vi "Tracking Test Teleop.vi"(10 "Match Info":T1={"Autonomous Elapsed Seconds"=0.0, "TeleOp Elapsed Seconds"=0.0, "Disabled Elapsed Seconds"=0.0, "Visited Autonomous"=FALSE, "Visited TeleOp"=FALSE, "Visited Disabled"=FALSE, "Autonomous Settings"={"Autonomous Style"=enum."Independent", "VI Refnum"=refnum}}, 11 "Call Context":T2) -> ()   [LabVIEW 2020]
doc: "This VI is called for each TeleOp packet received from the DS where the robot is not disabled. It is often used to read from the joysticks and update I/O or to update setpoints for timed control loops. It should complete and return within 20 milliseconds or it may miss DS packets."
uses:
  <vilib>/Rock Robotics/Network Tables/NT Write Boolean.vi
  Systems/Game Controller/Global_SEN_Data Out.vi
  Systems/Game Controller/GameController_SEN.lvlib
  Systems/SwerveDrive/Global_CMD_ACT_Data In.vi
  Systems/SwerveDrive/SwerveDrive_ACT.lvlib
  Shared Code/TypeDefs/ENUM_Swerve_CMD_Mode Select.ctl
  Shared Code/TypeDefs/Cluster_CMD_Direction Data.ctl
  Systems/SwerveDrive/Cluster_CMD_ACT_Data.ctl
  Shared Code/TypeDefs/Dial_Compase heading unit circle CCW positive.ctl
  Shared Code/TypeDefs/Level_Velocity plus-minus 1.ctl
  Shared Code/TypeDefs/Cluster_Module Velocity-Direction-Rotations.ctl
  Shared Code/TypeDefs/Cluster_X-Y.ctl
  <vilib>/Rock Robotics/WPI/ThirdParty/PhotonVisionLib/PhotonVisionLib.lvlib
  Type Defs/NUM_Rotate Input.ctl
  <vilib>/Rock Robotics/WPI/DriverStation/WPI_DriverStationMatch Info.ctl
  <vilib>/Rock Robotics/WPI/DriverStation/WPI_DriverStationDerivedRobotMode.ctl
panel:
  out "Rotation":dbl
  in  "Camera Pitch(deg)":dbl
  in  "TargetHeight_Meters":dbl=1.5
  in  "CameraHeight_Meters":dbl
  in  "CameraName":string="main"
  in  "Enabled":bool
  in  "Translation Speed (ft/s)":dbl=10.0 format="%#_13g"
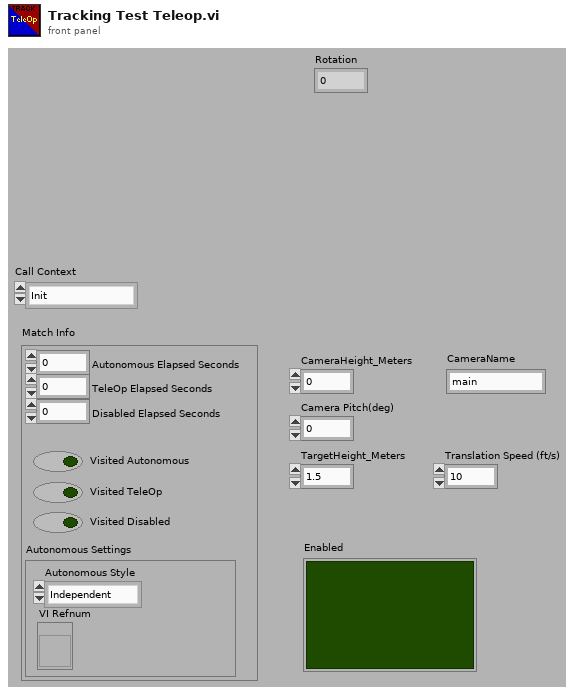
[diagram p1: front panel]
types:
  T1 = typedef "WPI_DriverStationMatch Info.ctl" = cluster{"Autonomous Elapsed Seconds":dbl, "TeleOp Elapsed Seconds":dbl, "Disabled Elapsed Seconds":dbl, "Visited Autonomous":bool, "Visited TeleOp":bool, "Visited Disabled":bool, "Autonomous Settings":cluster{"Autonomous Style":enum16{"Iterative", "Independent"}, "VI Refnum":refnum<vi>}}
  T2 = typedef "WPI_DriverStationDerivedRobotMode.ctl" = enum16{"Init", "Execute", "Stop"}
  T3 = typedef "Cluster_X-Y.ctl" = cluster{"X":dbl, "Y":dbl}
  T4 = typedef "ENUM_Swerve_CMD_Mode Select.ctl" = enum16{"Stop", "Move", "Turret Manual"}
  T5 = typedef "Cluster_Module Velocity-Direction-Rotations.ctl" = cluster{"Velocity":T6, "Angle":T7, "Rotations Count":dbl}
  T6 = typedef "Level_Velocity plus-minus 1.ctl" = dbl
  T7 = typedef "Dial_Compase heading unit circle CCW positive.ctl" = dbl
  T8 = typedef "SwerveDrive_ACT.lvlib/Cluster_CMD_ACT_Data.ctl" = cluster{"Mode":T4, "Direction":T9, "Orientation Robot(t) Field(f)":bool, "Max Translation Speed (ft/sec)":dbl, "Rotation Reduction 1-0":dbl, "Rotation Center From Robot Center":T3}
  T9 = typedef "Cluster_CMD_Direction Data.ctl" = cluster{"Traverse":T5, "Rotate(Yaw) CCW 1 CW -1":T10}
  T10 = typedef "NUM_Rotate Input.ctl" = dbl
  T11 = typedef "PhotonVisionLib.lvlib/PhotonPipelineResultType.ctl" = cluster{"TargetCount":i32, "Latency_MilliSec":dbl, "Targets":T12[]}
  T12 = typedef "PhotonVisionLib.lvlib/PhotonTrackedTargetType.ctl" = cluster{"Yaw":dbl, "Pitch":dbl, "Area":dbl, "Skew":dbl, "TargetCorners":T13[], "CameraToTarget":T14}
  T13 = typedef "PhotonVisionLib.lvlib/TargetCornerType.ctl" = cluster{"X":dbl, "Y":dbl}
  T14 = typedef "Trajectory_Library.lvlib/TRANSFORM2D.ctl" = cluster{"TRANSLATION":T15, "ROTATION":T16}
  T15 = typedef "Trajectory_Library.lvlib/TRANSLATION2D.ctl" = cluster{"X":dbl, "Y":dbl}
  T16 = typedef "Trajectory_Library.lvlib/ROTATION2D.ctl" = cluster{"VALUE":dbl, "COS":dbl, "SIN":dbl}
  T17 = typedef "Trajectory_Library.lvlib/ROTATION3D.ctl" = cluster{"Q_quaternion":T18}
  T18 = typedef "Trajectory_Library.lvlib/QUATERNION.ctl" = cluster{"R":dbl, "V":dbl[]}
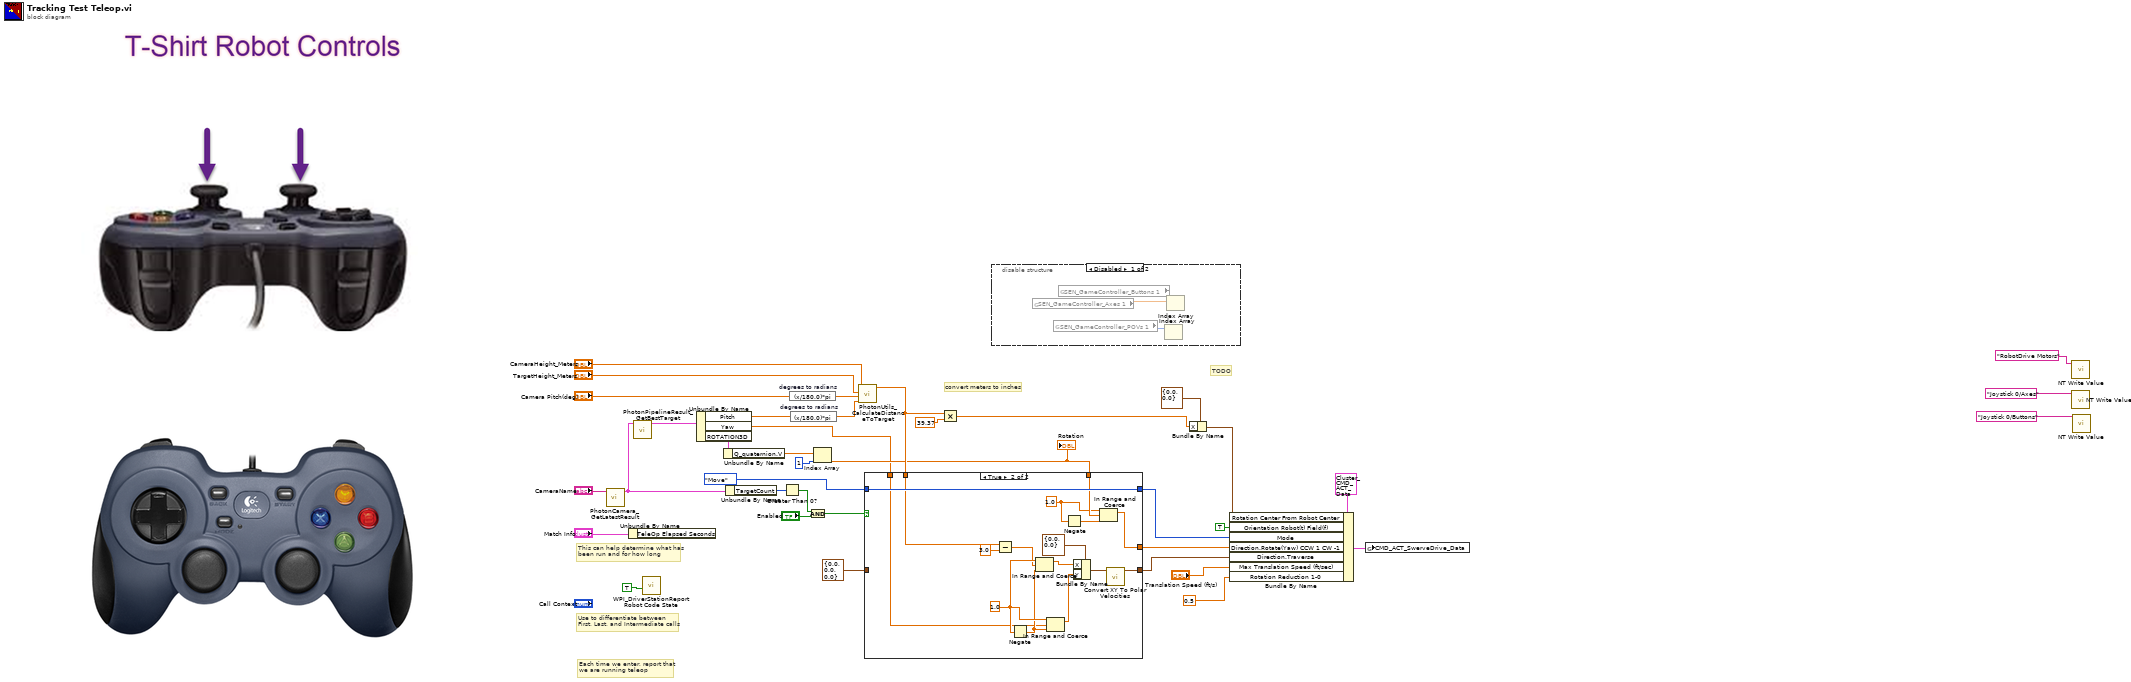
[diagram p0: block diagram]
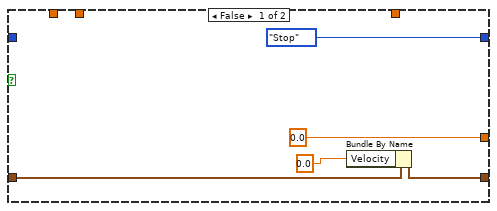
[diagram p2: hidden frame]
diagram:
  # "convert meters to inches"
  # "TODO"
  # "Each time we enter, report that\nwe are running teleop"
  # "Use to differentiate between\nFirst, Last, and Intermediate calls"
  # "This can help determine what has\nbeen run and for how long"
  n1 = call <vilib>:"PhotonCamera_GetLatestResult.vi"("CameraName"="CameraName") -> ("PipelineResult"=w19:T11)  [unwired: 9 in, 1 out]
  n2 = Unbundle By Name("Match Info") -> ()  [unwired: 1 out]
  n3 = call <vilib>:"PhotonPipelineResult_GetBestTarget.vi"("PhotonPipelineResult"=w19) -> ("PhotonTrackedTarget"=w6:T12)  [unwired: 10 in]
  n4 = call <vilib>:"WPI_DriverStationReport Robot Code State.vi"("TeleOp"=TRUE ("Autonomous")) -> ()  [unwired: 10 in, 1 out]
  n5 = Unbundle By Name(w6) -> ("Pitch"=w11:dbl, "Yaw"=w1:dbl, "ROTATION3D"=w4:T17)
  n6 = Unbundle By Name(w4) -> ("Q_quaternion.V"=w3:dbl[])
  n7 = Unbundle By Name(w19) -> ("TargetCount"=w23:i32)
  n8 = Greater Than 0?(x=w23) -> (x > 0?=w22:bool)
  n9 = expression code="(x/180.0)*pi" "degrees to radians"("Camera Pitch(deg)") -> (w15:dbl)
  n10 = expression code="(x/180.0)*pi" "degrees to radians"(w11) -> (w14:dbl)
  n11 = And(x=w22, y="Enabled") -> (x .and. y?=w20:bool)
  n12 = Index Array(array=w3, index=1) -> (element=w2:dbl)
  "Rotation" <- w2
  n13 = call <vilib>:"PhotonUtils_CalculateDistanceToTarget.vi"("TargetPitch_Radians"=w14, "CameraPitch_Radians"=w15, "TargetHeight_Meters"="TargetHeight_Meters", "CameraHeight_Meters"="CameraHeight_Meters") -> ("DistanceToTarget_Meters"=w9:dbl)  [unwired: 7 in]
  n14 = case shown="True" w20 {
    tunnel: ENUM_Swerve_CMD_Mode_Select."Move" ("Mode") -> [_ w59]
    tunnel: [ENUM_Swerve_CMD_Mode_Select."Stop" ("Mode") w59] -> w33
    tunnel: T5 {"Velocity"=0.0, "Angle"=0.0, "Rotations Count"=0.0} ("Polar Out") -> [w41 _]
    tunnel: [w42 w56] -> w29
    tunnel: w9 -> [_ w49]
    tunnel: w1 -> [_ w48]
    tunnel: [0.0 ("f") w44] -> w7
    tunnel: w2 -> [_ w47]
    frame False {
      n15 = Bundle By Name(cluster=w41, "Velocity"=T6 0.0) -> (w42:T5)
    }
    frame True {
      w45 = 1.0 ("upper limit")
      w54 = 1.0 ("upper limit")
      n16 = Subtract(x=w49, y=3.0) -> (x-y=w52:dbl)
      n17 = Negate(x=w54) -> (-x=w53:dbl)
      n18 = In Range and Coerce(upper limit=w54, x=w52, lower limit=w53) -> (coerced(x)=w51:dbl)  [unwired: 1 out]
      n19 = In Range and Coerce(upper limit=w54, x=w48, lower limit=w53) -> (coerced(x)=w50:dbl)  [unwired: 1 out]
      n20 = Negate(x=w45) -> (-x=w46:dbl)
      n21 = Bundle By Name(cluster=T3 {"X"=0.0, "Y"=0.0} ("XY Velocities"), "X"=w51, "Y"=w50) -> (w58:T3)
      n22 = In Range and Coerce(upper limit=w45, x=w47, lower limit=w46) -> (coerced(x)=w44:dbl)  [unwired: 1 out]
      n23 = call "Convert XY To Polar Velocities.vi"("XY Velocities"=w58) -> ("Polar Out"=w56:T5)  [unwired: 10 in]
    }
  }
  n24 = Multiply(x=w9, y=39.37) -> (x*y=w8:dbl)
  n25 = disable-structure shown="Disabled" {
    frame Disabled {
      n26 = global read "Global_SEN_Data Out.vi" "SEN_GameController_Axes 1"() -> (w61:dbl[])
      n27 = global read "Global_SEN_Data Out.vi" "SEN_GameController_POVs 1"() -> (w60:i16[])
      n28 = global read "Global_SEN_Data Out.vi" "SEN_GameController_Buttons 1"() -> ()  [unwired: 1 out]
      n29 = Index Array(array=w60) -> ()  [unwired: 1 in, 1 out]
      n30 = Index Array(array=w61) -> ()  [unwired: 1 in, 1 out]
    }
    frame Enabled {
    }
  }
  n31 = Bundle By Name(cluster=T3 {"X"=0.0, "Y"=0.0} ("Rotation Center From Robot Center"), "X"=w8) -> (w17:T3)
  n32 = Bundle By Name(cluster=T8 {"Mode"=enum."Stop", "Direction"={"Traverse"={"Velocity"=0.0, "Angle"=0.0, "Rotations Count"=0.0}, "Rotate(Yaw) CCW 1 CW -1"=0.0}, "Orientation Robot(t) Field(f)"=FALSE, "Max Translation Speed (ft/sec)"=0.0, "Rotation Reduction 1-0"=0.0, "Rotation Center From Robot Center"={"X"=0.0, "Y"=0.0}} ("CMD_ACT_Template_Data"), "Rotation Center From Robot Center"=w17, "Orientation Robot(t) Field(f)"=TRUE, "Mode"=w33, "Direction.Rotate(Yaw) CCW 1 CW -1"=w7, "Direction.Traverse"=w29, "Max Translation Speed (ft/sec)"="Translation Speed (ft/s)", "Rotation Reduction 1-0"=0.5) -> (w31:T8)
  n33 = global write "Global_CMD_ACT_Data In.vi" "CMD_ACT_SwerveDrive_Data"(w31) -> ()
  n34 = call-poly <vilib>:"NT Write Value.vi"("name"="RobotDrive Motors" ("Name")) -> ()  [unwired: 10 in, 1 out]
  n35 = call-poly <vilib>:"NT Write Value.vi"("name"="Joystick 0/Axes" ("Name")) -> ()  [unwired: 10 in, 1 out]
  n36 = call-poly <vilib>:"NT Write Value.vi"("name"="Joystick 0/Buttons" ("Name")) -> ()  [unwired: 10 in, 1 out]
